vi "XNET Create Session (Generic).vi"(5 "list (empty)":string[](array[string]), 7 "mode":T1 items=["Signal Input Single-point", "Signal Input Waveform", "Signal Input XY", "Signal Output Single-point", "Signal Output Waveform", "Signal Output XY", "Frame Input Stream", "Frame Input Queued", "Frame Input Single-point", "Frame Output Stream", "Frame Output Queued", "Frame Output Single-point", "Conversion"], 9 "interface":refnum<k21>, 11 "error in (no error)":errorcluster, 12 "database (:memory:)":string=":memory:", 13 "cluster (empty)":string) -> (4 "session out":refnum<k21>, 15 "error out":errorcluster)   [LabVIEW 2018]
doc: "Creates an XNET session at run time using strings instead of XNET I/O names. This VI is for advanced applications, when you need to store the configuration as strings (such as within a text file)."
uses:
  XNET Mode.ctl
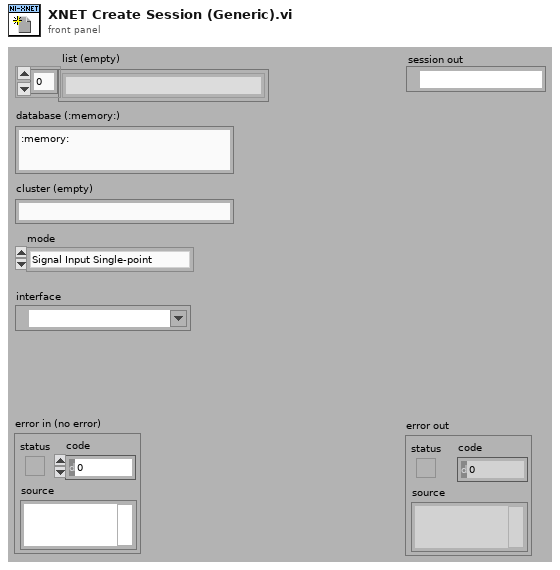
[diagram p1: front panel]
types:
  T1 = typedef "XNET Mode.ctl" = u32
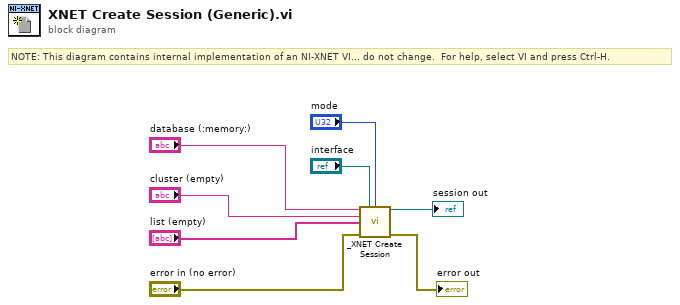
[diagram p0: block diagram]
diagram:
  # "NOTE: This diagram contains internal implementation of an NI-XNET VI... do not change.  For help, select VI and press Ctrl-H."
  n1 = call "_XNET Create Session.vi"("database (empty)"="database (:memory:)", "interface"="interface", "mode"="mode", "cluster (empty)"="cluster (empty)", "signal/frame list (empty)"="list (empty)", "error in (no error)"="error in (no error)") -> ("session out"=→"session out":refnum<k21>, "error out"=→"error out":errorcluster)  [unwired: 8 out]
